vi "Read Name core.vi"(11 "Build Item in":refnum<class "Build VIPB Step.lvclass">) -> (2 "Name":string)   [LabVIEW 2019, in "VIPM.lvlib" / "Build VIPB Step.lvclass"]
doc: "Gets the name for the build step\n\nCopyright: MGI 2016\nAuthor: Derek Trepanier"
uses:
  Build VIPB Step.lvclass
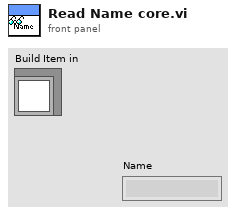
[diagram p1: front panel]
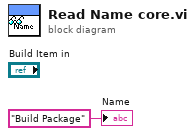
[diagram p0: block diagram]
diagram:
  "Name" <- "Build Package" ("Name")
